vi "Make_Settings_Item.vi"(8 "error in (no error)":errorcluster, 10 "address":string[](array[string]), 11 "IB_Source_File in":refnum<class "IB_Source_File.lvclass">) -> (0 "error out":errorcluster, 3 "IB_Settings_Item.lvclass":refnum<class "IB_Settings_Item.lvclass">)   [LabVIEW 2020, in "IB_Source_File.lvclass"]
uses:
  <vilib>/AppBuilder/IB_Classes/Source/File/IB_Source_File.lvclass
  <vilib>/AppBuilder/IB_Classes/Source/File/IB_Source_File.lvclass/IB_Source_File.ctl
  <vilib>/AppBuilder/IB_Classes/Settings_Item_File/IB_Settings_Item_File.lvclass
  <vilib>/AppBuilder/IB_Classes/Settings_Item/IB_Settings_Item.lvclass
  e:/builds/penguin/labview/branches/2020/dev/dist/vi.lib/AppBuilder/IB_Classes/Settings_Item/IB_Settings_Item.lvclass
  e:/builds/penguin/labview/branches/2020/dev/dist/vi.lib/AppBuilder/IB_Classes/Settings_Item_File/IB_Settings_Item_File.lvclass
  e:/builds/penguin/labview/branches/2020/dev/dist/vi.lib/AppBuilder/IB_Classes/Source/IB_Source.lvclass
  e:/builds/penguin/labview/branches/2020/dev/dist/vi.lib/AppBuilder/IB_Classes/Source/File/IB_Source_File.lvclass
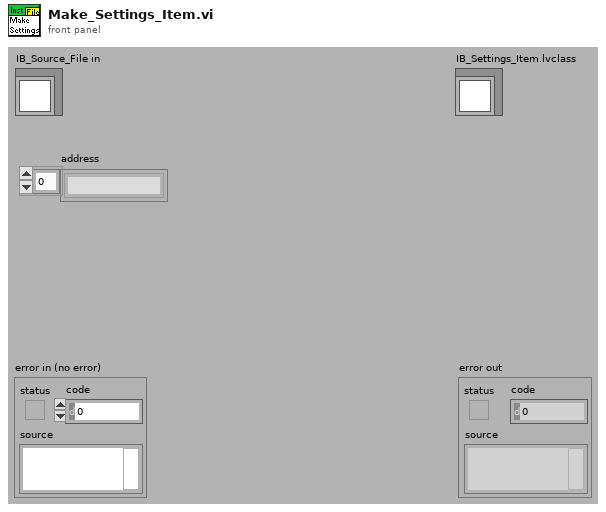
[diagram p1: front panel]
types:
  T1 = typedef "IB_Settings_Item.ctl" = cluster{"address":string[], "Attributes":i16, "RegCOM":bool, "unlock":bool}
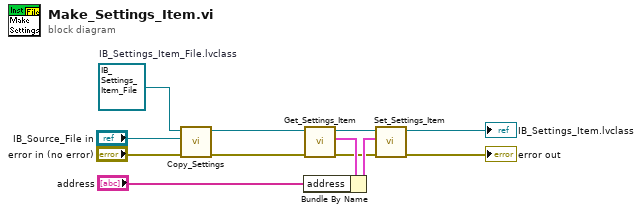
[diagram p0: block diagram]
diagram:
  w11 = refnum<class "IB_Settings_Item_File.lvclass"> refnum  # IB_Settings_Item_File.lvclass
  n1 = call-dynamic "Copy_Settings.vi"("error in (no error)"="error in (no error)", "LabVIEW Object"="IB_Source_File in", "IB_Settings_Item_File in"=w11) -> ("error out"=w3:errorcluster, "IB_Settings_Item_File out"=w8:refnum<class "IB_Settings_Item_File.lvclass">)  [unwired: 7 in]
  n2 = call <vilib>:"Get_Settings_Item.vi"("error in (no error)"=w3, "IB_Settings_Item in"=w8) -> ("error out"=w4:errorcluster, "data"=w6:T1, "IB_Settings_Item out"=w9:refnum<class "IB_Settings_Item_File.lvclass">)  [unwired: 7 in]
  n3 = Bundle By Name(cluster=w6, "address"="address") -> (w5:T1)
  n4 = call <vilib>:"Set_Settings_Item.vi"("error in (no error)"=w4, "data"=w5, "IB_Settings_Item in"=w9) -> ("error out"=→"error out":errorcluster, "IB_Settings_Item out"=→"IB_Settings_Item.lvclass":refnum<class "IB_Settings_Item_File.lvclass">)  [unwired: 7 in]
